vi "USBImage.vi"() -> ()   [LabVIEW 2015]
panel:
  out "Intensity Graph":i32[][](graph)
  out "Set Image":u32
  out "Set Gate Mode":u32
  out "Shut Down":u32
  out "Detector Y Pixels":i32
  out "Get Detector":u32
  out "Get Status":u32
  out "Set Exposure Time":u32
  out "Set Trigger Mode":u32
  out "Set Readout Mode":u32
  out "Set Acquisition Mode":u32
  out "Check Timings":u32
  out "Detector X Pixels":i32
  out "Status":u32
  out "Start Acquisition":u32
  out "Get Acquired Data":u32
  out "Calculated Exposure Value":sgl format="%.5f"
  in  "Exposure Time (secs)":sgl format="%.2f"
  out "Initialize":u32
  in  "Trigger":u32(ring) items=["Internal", "External"]
  # "Status"
  # "Return values"
  # "USB iStarIMAG32at.VI"
  # "Acquisition Mode: Single Scan\nReadout Mode: Full Resolution Image"
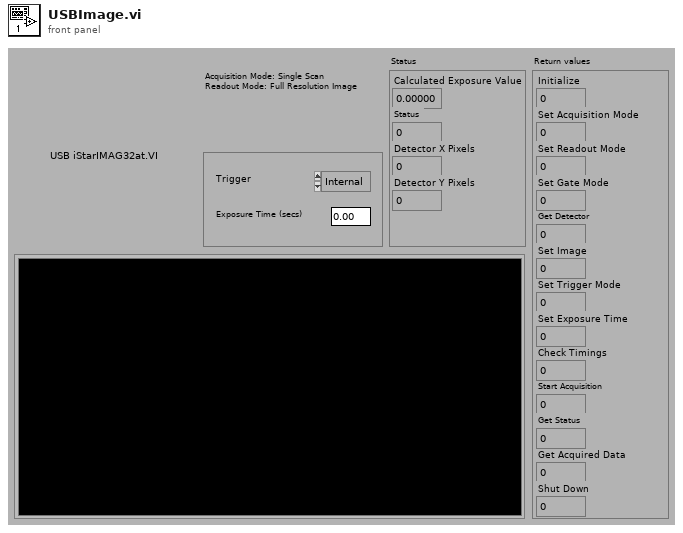
[diagram p1: front panel]
types:
  T1 = typedef "Error Code Enum typedef.ctl" = enum32{"N/A (0)", "DRV_ERROR_CODES", "DRV_SUCCESS", "DRV_VXDNOTINSTALLED", "DRV_ERROR_SCAN", "DRV_ERROR_CHECK_SUM", "DRV_ERROR_FILELOAD", "DRV_UNKNOWN_FUNC", "DRV_ERROR_VXD_INIT", "DRV_ERROR_ADDRESS", "DRV_ERROR_PAGELOCK", "DRV_ERROR_PAGEUNLOCK", "DRV_ERROR_BOARDTEST", "DRV_ERROR_ACK", "DRV_ERROR_UP_FIFO", "DRV_ERROR_PATTERN", "N/A (16)", "DRV_ACQUISITION_ERRORS", "DRV_ACQ_BUFFER", "DRV_ACQ_DOWNFIFO_FULL", "DRV_PROC_UNKONWN_INSTRUCTION", "DRV_ILLEGAL_OP_CODE", "DRV_KINETIC_TIME_NOT_MET", "DRV_ACCUM_TIME_NOT_MET", "DRV_NO_NEW_DATA", "N/A (25)", "DRV_SPOOLERROR", "N/A (27)", "N/A (28)", "N/A (29)", "N/A (30)", "N/A (31)", "N/A (32)", "DRV_TEMPERATURE_CODES", "DRV_TEMPERATURE_OFF", "DRV_TEMPERATURE_NOT_STABILIZED", "DRV_TEMPERATURE_STABILIZED", "DRV_TEMPERATURE_NOT_REACHED", "DRV_TEMPERATURE_OUT_RANGE", "DRV_TEMPERATURE_NOT_SUPPORTED", "DRV_TEMPERATURE_DRIFT", "N/A (41)", "N/A (42)", "N/A (43)", "N/A (44)", "N/A (45)", "N/A (46)", "N/A (47)", "N/A (48)", "DRV_GENERAL_ERRORS", "DRV_INVALID_AUX", "DRV_COF_NOTLOADED", "DRV_FPGAPROG", "DRV_FLEXERROR", "DRV_GPIBERROR", "N/A (55)", "N/A (56)", "N/A (57)", "N/A (58)", "N/A (59)", "N/A (60)", "N/A (61)", "N/A (62)", "N/A (63)", "DRV_DATATYPE", "DRV_DRIVER_ERRORS", "DRV_P1INVALID", "DRV_P2INVALID", "DRV_P3INVALID", "DRV_P4INVALID", "DRV_INIERROR", "DRV_COFERROR", "DRV_ACQUIRING", "DRV_IDLE", "DRV_TEMPCYCLE", "DRV_NOT_INITIALIZED", "DRV_P5INVALID", "DRV_P6INVALID", "DRV_INVALID_MODE", "DRV_INVALID_FILTER", "DRV_I2CERRORS", "DRV_I2CDEVNOTFOUND", "DRV_I2CTIMEOUT", "DRV_P7INVALID", "N/A (84)", "N/A (85)", "N/A (86)", "N/A (87)", "N/A (88)", "N/A (89)", "DRV_IOCERROR", "DRV_VRMVERSIONERROR"}
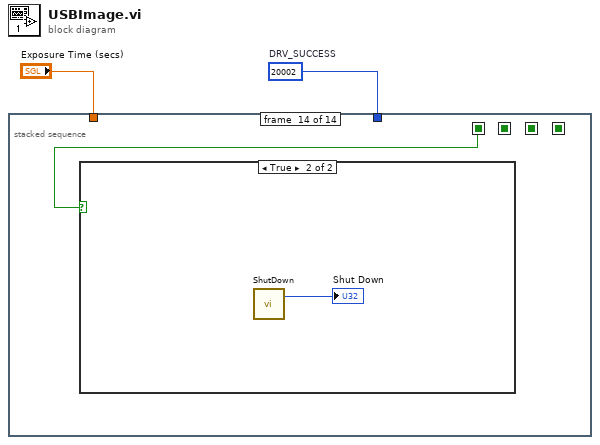
[diagram p0: block diagram]
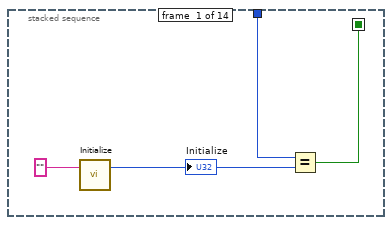
[diagram p2: hidden frame]
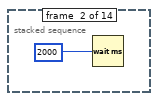
[diagram p3: hidden frame]
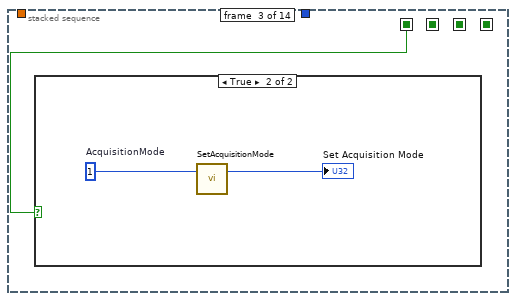
[diagram p4: hidden frame]
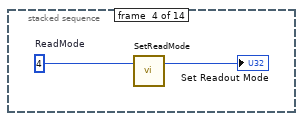
[diagram p6: hidden frame]
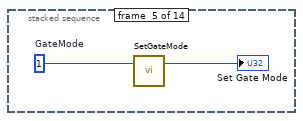
[diagram p7: hidden frame]
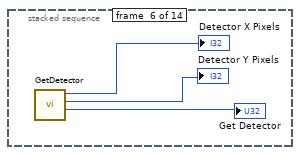
[diagram p8: hidden frame]
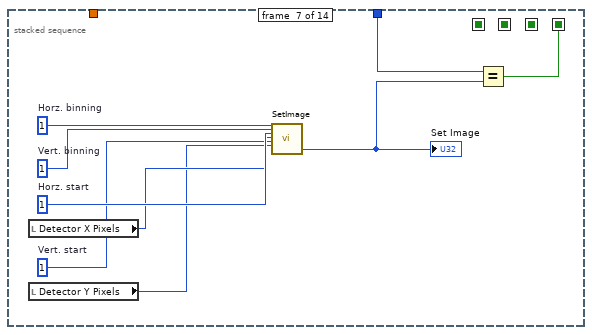
[diagram p9: hidden frame]
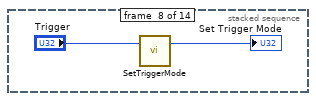
[diagram p10: hidden frame]
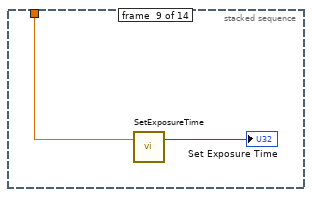
[diagram p11: hidden frame]
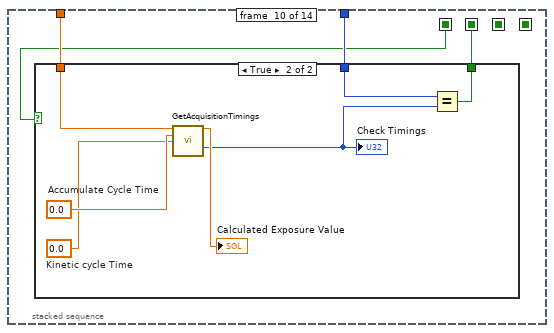
[diagram p12: hidden frame]
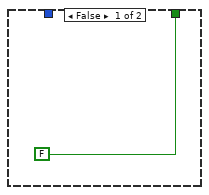
[diagram p13: hidden frame]
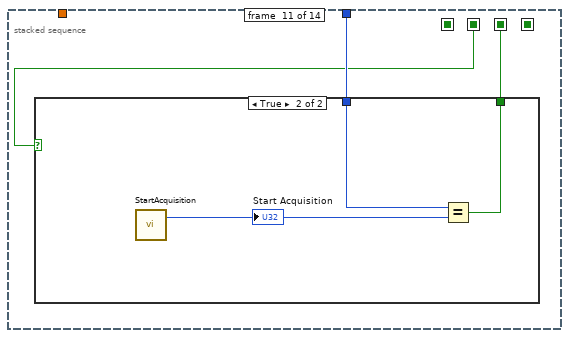
[diagram p14: hidden frame]
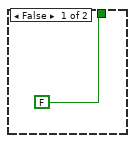
[diagram p15: hidden frame]
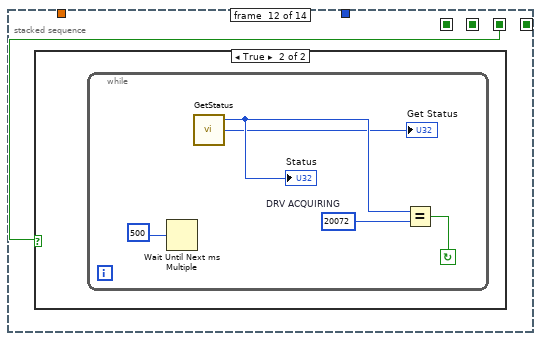
[diagram p16: hidden frame]
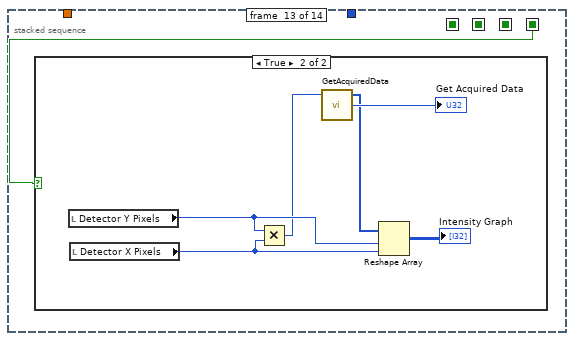
[diagram p18: hidden frame]
diagram:
  w1 = 20002  # DRV_SUCCESS
  n1 = stacked-sequence {
    seq-local: [w5 _ _ _ _ _ _ _ _ _ _ _ _ _] -> [_ _ w8 _ _ _ _ _ _ w31 _ _ _ w63]
    seq-local: [_ _ _ _ _ _ _ _ _ w32 _ _ _ _] -> [_ _ _ _ _ _ _ _ _ _ w44 _ _ _]
    seq-local: [_ _ _ _ _ _ _ _ _ _ w43 _ _ _] -> [_ _ _ _ _ _ _ _ _ _ _ w50 _ _]
    seq-local: [_ _ _ _ _ _ w24 _ _ _ _ _ _ _] -> [_ _ _ _ _ _ _ _ _ _ _ _ w56 _]
    tunnel: "Exposure Time (secs)" -> [_ _ _ _ _ _ _ _ w30 w34 _ _ _ _]
    tunnel: w1 -> [w6 _ _ _ _ _ w26 _ _ w33 w45 _ _ _]
    frame #0 {
      n2 = call "Initialize.vi"("directory (\"\")"="") -> ("DLL error code"=w3:u32)  [unwired: 1 in, 1 out]
      "Initialize" <- w3
      n3 = Equal?(x=w6, y=w3) -> (x = y?=w5:bool)
    }
    frame #1 {
      n4 = Wait (ms)(milliseconds to wait=u32 2000) -> ()  [unwired: 1 out]
    }
    frame #2 {
      n5 = case shown="True" w8 {
        frame False {
        }
        frame True {
          w10 = u16 1  # AcquisitionMode
          n6 = call "SetAcquisitionMode.vi"("mode"=w10) -> ("DLL error code"=→"Set Acquisition Mode":u32)  [unwired: 1 in, 1 out]
        }
      }
    }
    frame #3 {
      w11 = u16 4  # ReadMode
      n7 = call "SetReadMode.vi"("mode"=w11) -> ("DLL error code"=→"Set Readout Mode":u32)  [unwired: 1 in, 1 out]
    }
    frame #4 {
      w13 = u16 1  # GateMode
      n8 = call "SetGateMode.vi"("mode"=w13) -> ("DLL error code"=→"Set Gate Mode":u32)  [unwired: 1 in, 1 out]
    }
    frame #5 {
      n9 = call "GetDetector.vi"() -> ("DLL error code"=→"Get Detector":u32, "ypixels"=→"Detector Y Pixels":i32, "xpixels"=→"Detector X Pixels":i32)  [unwired: 4 in, 1 out]
    }
    frame #6 {
      w19 = u16 1  # Vert. start
      w22 = u16 1  # Horz. start
      w21 = u16 1  # Vert. binning
      w23 = u16 1  # Horz. binning
      n10 = local read "Detector X Pixels"() -> (w20:i32)
      n11 = local read "Detector Y Pixels"() -> (w18:i32)
      n12 = call "SetImage.vi"("hbin"=w23, "vbin"=w21, "hstart"=w22, "hend"=w20, "vstart"=w19, "vend"=w18) -> ("DLL error code"=w25:u32)  [unwired: 20 in, 1 out]
      "Set Image" <- w25
      n13 = Equal?(x=w26, y=w25) -> (x = y?=w24:bool)
    }
    frame #7 {
      n14 = call "SetTriggerMode.vi"("mode"="Trigger") -> ("DLL error code"=→"Set Trigger Mode":u32)  [unwired: 1 in, 1 out]
    }
    frame #8 {
      n15 = call "SetExposureTime.vi"("time"=w30) -> ("DLL error code"=→"Set Exposure Time":u32)  [unwired: 1 in, 1 out]
    }
    frame #9 {
      n16 = case shown="True" w31 {
        tunnel: w34 -> [_ w40]
        tunnel: w33 -> [_ w41]
        tunnel: [FALSE w42] -> w32
        frame False {
        }
        frame True {
          w39 = sgl 0.0  # Accumulate Cycle Time
          w38 = sgl 0.0  # Kinetic cycle Time
          n17 = call "GetAcquisitionTimings.vi"("exposure input"=w40, "accumulate input"=w39, "kinetic input"=w38) -> ("exposure"=→"Calculated Exposure Value":sgl, "DLL error code"=w36:u32)  [unwired: 8 in, 3 out]
          "Check Timings" <- w36
          n18 = Equal?(x=w41, y=w36) -> (x = y?=w42:bool)
        }
      }
    }
    frame #10 {
      n19 = case shown="True" w44 {
        tunnel: [FALSE w49] -> w43
        tunnel: w45 -> [_ w48]
        frame False {
        }
        frame True {
          n20 = call "StartAcquisition.vi"() -> ("DLL error code"=w47:u32)  [unwired: 2 in, 1 out]
          "Start Acquisition" <- w47
          n21 = Equal?(x=w48, y=w47) -> (x = y?=w49:bool)
        }
      }
    }
    frame #11 {
      n22 = case shown="True" w50 {
        frame False {
        }
        frame True {
          n23 = while {
            stop <- w54 continue-if-true
            w53 = u16 20072  # DRV ACQUIRING
            n24 = Wait Until Next ms Multiple(millisecond multiple=u32 500) -> ()  [unwired: 1 out]
            n25 = call "GetStatus.vi"() -> ("DLL error code"=→"Get Status":u32, "status"=w52:T1)  [unwired: 3 in, 1 out]
            "Status" <- w52
            n26 = Equal?(x=w52, y=w53) -> (x = y?=w54:bool)
          }
        }
      }
    }
    frame #12 {
      n27 = case shown="True" w56 {
        frame False {
        }
        frame True {
          n28 = local read "Detector Y Pixels"() -> (w60:i32)
          n29 = local read "Detector X Pixels"() -> (w59:i32)
          n30 = Multiply(x=w60, y=w59) -> (x*y=w58:i32)
          n31 = call "GetAcquiredData.vi"("size"=w58) -> ("DLL error code"=→"Get Acquired Data":u32, "array"=w57:i32[])  [unwired: 2 in, 1 out]
          n32 = Reshape Array(w57, w60, w59) -> (→"Intensity Graph":i32[][])
        }
      }
    }
    frame #13 {
      n33 = case shown="True" w63 {
        frame False {
        }
        frame True {
          n34 = call "ShutDown.vi"() -> ("DLL error code"=→"Shut Down":u32)  [unwired: 2 in, 1 out]
        }
      }
    }
  }
